vi "Dispatch Tx.vi"(8 "error in (no error)":errorcluster, 9 "framework iteration":u64, 10 "Dispatcher Interface in":refnum<class "Dispatcher Interface.lvclass">, 11 "Scheduler in":refnum<class "Scheduler.lvclass">) -> (0 "error out":errorcluster, 2 "Dispatcher Interface out":refnum<class "Dispatcher Interface.lvclass">, 3 "Scheduler out":refnum<class "Scheduler.lvclass">)   [LabVIEW 2017, in "DSF Core.lvlib" / "Scheduler.lvclass"]
uses:
  Scheduler.lvclass
  Interfaces/Dispatcher/Dispatcher Interface.lvclass
  Interfaces/Dispatcher/Command.ctl
  Scheduler.lvclass/Scheduler.ctl
  Scheduler Plugin Bundle.lvclass
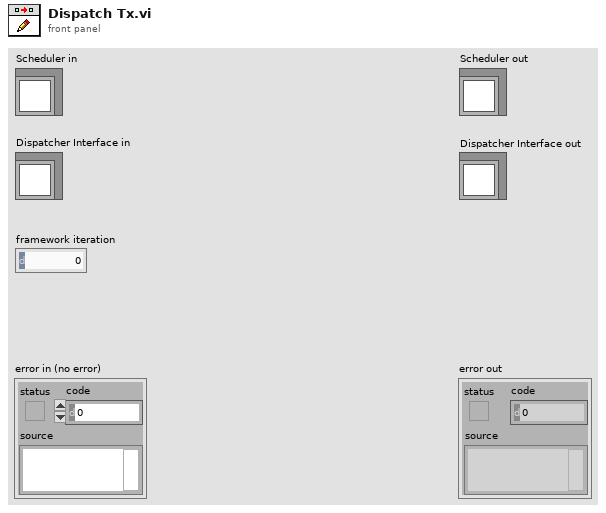
[diagram p1: front panel]
types:
  T1 = typedef "DSF Core.lvlib/Dispatcher Interface.lvclass/Command.ctl" = enum8{"Rx", "Tx", "Shutdown"}
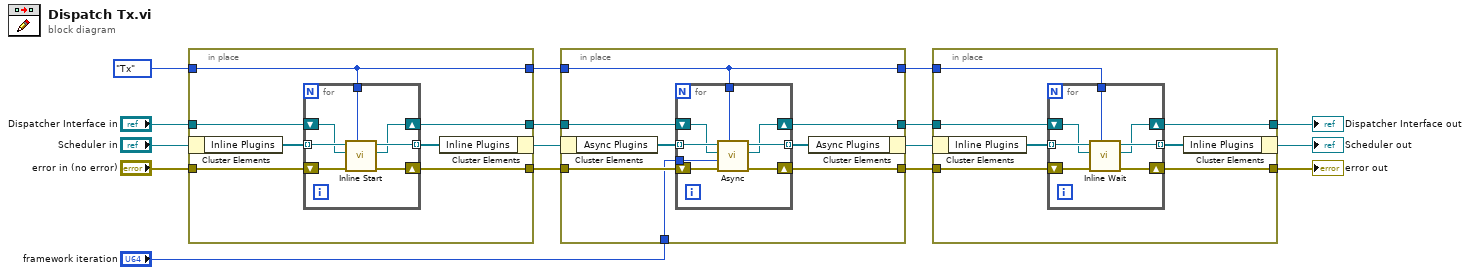
[diagram p0: block diagram]
diagram:
  n1 = in-place {
    in-place-border: "Dispatcher Interface in" -> [w22]
    in-place-border: [w21] -> w12
    in-place-border: "error in (no error)" -> [w20]
    in-place-border: [w19] -> w13
    in-place-border: Command."Tx" ("command") -> [w17]
    in-place-border: [w17] -> w2
    n2 = in-place-cluster #1("Scheduler in") -> ("Inline Plugins"=w23:refnum<class "Scheduler Plugin Bundle.lvclass">[])
    n3 = for {
      tunnel: w23 -> [w27] mode=indexing
      shift-right: [w28] -> w21
      shift-left: w22 -> [w26]
      shift-right: [w25] -> w19
      shift-left: w20 -> [w30]
      tunnel: [w29] -> w18 mode=indexing
      tunnel: w17 -> [w24]
      n4 = call "Inline Start.vi"("Command"=w24, "error in (no error)"=w30, "Dispatcher Interface in"=w26, "Plugin Timing Group in"=w27) -> ("error out"=w25:errorcluster, "Dispatcher Interface out"=w28:refnum<class "Dispatcher Interface.lvclass">, "Plugin Timing Group out"=w29:refnum<class "Scheduler Plugin Bundle.lvclass">)  [unwired: 5 in]
    }
    n5 = in-place-cluster #1("Inline Plugins"=w18) -> (w11:refnum<class "Scheduler.lvclass">)
  }
  n6 = in-place {
    in-place-border: w12 -> [w37]
    in-place-border: [w36] -> w8
    in-place-border: w13 -> [w35]
    in-place-border: [w34] -> w10
    in-place-border: "framework iteration" -> [w32]
    in-place-border: w2 -> [w31]
    in-place-border: [w31] -> w1
    n7 = in-place-cluster #2(w11) -> ("Async Plugins"=w38:refnum<class "Scheduler Plugin Bundle.lvclass">[])
    n8 = for {
      tunnel: w38 -> [w42] mode=indexing
      shift-right: [w43] -> w36
      shift-left: w37 -> [w41]
      shift-right: [w46] -> w34
      shift-left: w35 -> [w45]
      tunnel: [w44] -> w33 mode=indexing
      tunnel: w32 -> [w40]
      tunnel: w31 -> [w39]
      n9 = call "Async.vi"("command"=w39, "error in (no error)"=w45, "framework iteration"=w40, "Dispatcher Interface in"=w41, "Plugin Timing Bundle in"=w42) -> ("error out"=w46:errorcluster, "Dispatcher Interface out"=w43:refnum<class "Dispatcher Interface.lvclass">, "Plugin Timing Bundle out"=w44:refnum<class "Scheduler Plugin Bundle.lvclass">)  [unwired: 4 in]
    }
    n10 = in-place-cluster #2("Async Plugins"=w33) -> (w9:refnum<class "Scheduler.lvclass">)
  }
  n11 = in-place {
    in-place-border: w8 -> [w52]
    in-place-border: [w51] -> w5
    in-place-border: w10 -> [w50]
    in-place-border: [w49] -> w6
    in-place-border: w1 -> [w47]
    n12 = in-place-cluster #3(w9) -> ("Inline Plugins"=w53:refnum<class "Scheduler Plugin Bundle.lvclass">[])
    n13 = for {
      tunnel: w53 -> [w56] mode=indexing
      shift-right: [w57] -> w51
      shift-left: w52 -> [w55]
      shift-right: [w60] -> w49
      shift-left: w50 -> [w59]
      tunnel: [w58] -> w48 mode=indexing
      tunnel: w47 -> [w54]
      n14 = call "Inline Wait.vi"("Command"=w54, "error in (no error)"=w59, "Dispatcher Interface in"=w55, "Plugin Timing Group in"=w56) -> ("error out"=w60:errorcluster, "Dispatcher Interface out"=w57:refnum<class "Dispatcher Interface.lvclass">, "Plugin Timing Group out"=w58:refnum<class "Scheduler Plugin Bundle.lvclass">)  [unwired: 5 in]
    }
    n15 = in-place-cluster #3("Inline Plugins"=w48) -> (→"Scheduler out":refnum<class "Scheduler.lvclass">)
  }
  "error out" <- w6
  "Dispatcher Interface out" <- w5
